vi "CreateRollingAverage.vi"(8 "Error In":errorcluster, 10 "Example Value":dbl=nan, 11 "Number of Points":i32=10) -> (0 "Error Out":errorcluster, 3 "Rolling Average Queue Out":refnum<queue>)   [LabVIEW 2012, in "LV-Utilities.lvlib"]
uses:
  LV-Utilities.lvlib
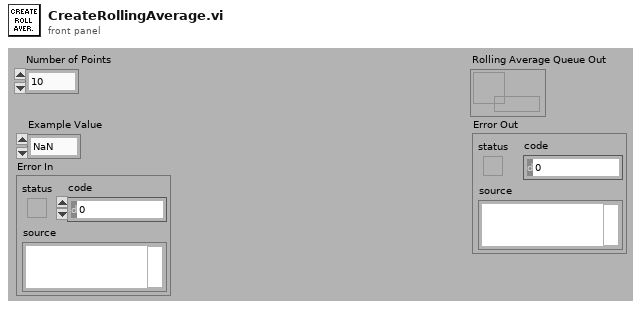
[diagram p1: front panel]
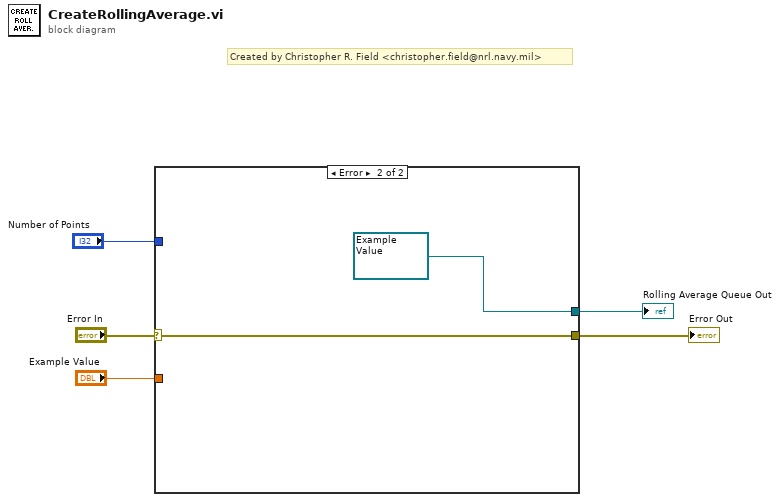
[diagram p0: block diagram]
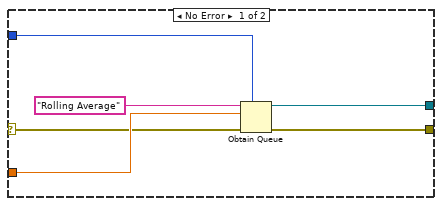
[diagram p2: hidden frame]
diagram:
  # "Created by Christopher R. Field <christopher.field@nrl.navy.mil>"
  n1 = case shown="Error" "Error In" {
    selector: "Error In" -> [w6 w13]
    tunnel: [w10 refnum<queue> refnum ("queue out")] -> w3
    tunnel: [w9 w13] -> w5
    tunnel: "Example Value" -> [w8 _]
    tunnel: "Number of Points" -> [w7 _]
    frame No Error {
      n2 = Obtain Queue(max queue size (-1, unlimited)=w7, name (unnamed)="Rolling Average", element data type=w8, error in (no error)=w6) -> (queue out=w10:refnum<queue>, error out=w9:errorcluster)  [unwired: 1 in, 1 out]
    }
    frame Error {
    }
  }
  "Rolling Average Queue Out" <- w3
  "Error Out" <- w5
